vi "Adjust Font Size to Rectangle.vi"(7 "String Control Reference":refnum<vi>, 8 "Message":string, 9 "Bold?":bool, 10 "Maximum Size (45)":i16=45, 11 "Minimum Size (15)":i16=15) -> (3 "Font Size":u32)   [LabVIEW 2015, in "Test Class.lvclass"]
uses:
  Test Class.lvclass
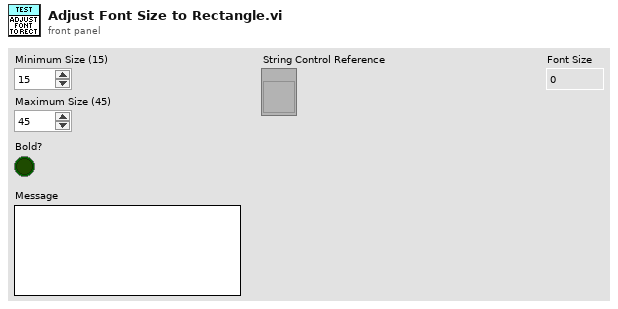
[diagram p1: front panel]
types:
  T1 = cluster{"Font Name:":string, "Size":i16, "Strikeout?":bool, "Italic?":bool, "Underline?":bool, "Outline?":bool, "Shadow?":bool, "Bold?":bool}
  T2 = enum16{"User-specified Font", "Application Font", "System Font", "Dialog Font"}
  T3 = cluster{"left":i16, "top":i16, "right":i16, "bottom":i16}
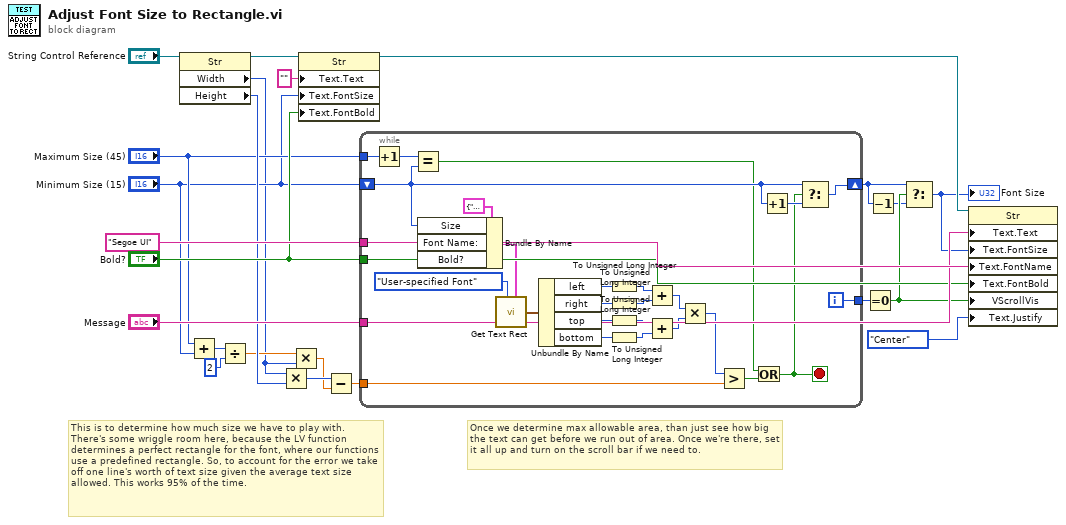
[diagram p0: block diagram]
diagram:
  w23 = "Segoe UI" ("Font Name:")
  # "Once we determine max allowable area, than just see how big the text can get before we run out of area. Once we're there, set it all up and turn on the scroll bar if we need to."
  # "This is to determine how much size we have to play with. There's some wriggle room here, because the LV function determines a perfect rectangle for the font, where our functions use a predefined rectangle. So, to account for the error we take off one line's worth of text size given the average text size allowed. This works 95% of the time."
  n1 = property on="Property Node" class="Str"(reference="String Control Reference") -> (reference out=w13:refnum<vi>, "Width"=w1:u32, "Height"=w11:u32)  [unwired: 1 in, 1 out]
  n2 = Add(x="Maximum Size (45)", y="Minimum Size (15)") -> (x+y=w6:i16)
  n3 = Divide(x=w6, y=i16 2) -> (x/y=w4:dbl)
  n4 = Multiply(x=w1, y=w11) -> (x*y=w18:u32)
  n5 = Multiply(x=w4, y=w1) -> (x*y=w17:dbl)
  n6 = property on="Property Node" class="Str"(reference=w13, "Text.Text"="", "Text.FontSize"="Minimum Size (15)", "Text.FontBold"="Bold?") -> (reference out=w12:refnum<vi>)  [unwired: 1 in, 1 out]
  n7 = Subtract(x=w18, y=w17) -> (x-y=w16:dbl)
  n8 = while {
    tunnel: "Message" -> [w50]
    tunnel: w23 -> [w48]
    tunnel: "Bold?" -> [w47]
    shift-right: [w30] -> w7
    shift-left: "Minimum Size (15)" -> [w28]
    tunnel: w16 -> [w41]
    tunnel: [w39] -> w22
    tunnel: "Maximum Size (45)" -> [w29]
    i -> [w39]
    stop <- w25 stop-if-true
    n9 = Increment(x=w29) -> (x+1=w24:i16)
    n10 = Equal?(x=w24, y=w28) -> (x = y?=w26:bool)
    n11 = Bundle By Name(cluster=T1 {"Font Name:"="Segoe UI", "Size"=0, "Strikeout?"=FALSE, "Italic?"=FALSE, "Underline?"=FALSE, "Outline?"=FALSE, "Shadow?"=FALSE, "Bold?"=FALSE} ("[user-specified font]"), "Size"=w28, "Font Name:"=w48, "Bold?"=w47) -> (w46:T1)
    n12 = call <vilib>:"Get Text Rect.vi"("desired font(Application)"=T2."User-specified Font", "text"=w50, "[user-specified font]"=w46) -> ("rect"=w45:T3)  [unwired: 6 in]
    n13 = Unbundle By Name(w45) -> ("left"=w44:i16, "right"=w38:i16, "top"=w37:i16, "bottom"=w36:i16)
    n14 = To Unsigned Long Integer(number=w44) -> (unsigned 32bit integer=w33:u32)
    n15 = To Unsigned Long Integer(number=w38) -> (unsigned 32bit integer=w32:u32)
    n16 = To Unsigned Long Integer(number=w37) -> (unsigned 32bit integer=w35:u32)
    n17 = To Unsigned Long Integer(number=w36) -> (unsigned 32bit integer=w34:u32)
    n18 = Add(x=w33, y=w32) -> (x+y=w42:u32)
    n19 = Add(x=w35, y=w34) -> (x+y=w43:u32)
    n20 = Multiply(x=w42, y=w43) -> (x*y=w40:u32)
    n21 = Greater?(x=w40, y=w41) -> (0:w27:bool)
    n22 = Or(x=w26, y=w27) -> (x .or. y?=w25:bool)
    n23 = Increment(x=w28) -> (x+1=w31:i16)
    n24 = Select(t=w28, s=w25, f=w31) -> (s? t:f=w30:i16)
  }
  n25 = Equal To 0?(x=w22) -> (x = 0?=w9:bool)
  n26 = Decrement(x=w7) -> (x-1=w8:i16)
  n27 = Select(t=w7, s=w9, f=w8) -> (s? t:f=w10:i16)
  "Font Size" <- w10
  n28 = property on="Property Node" class="Str"(reference=w12, "Text.Text"="Message", "Text.FontSize"=w10, "Text.FontName"=w23, "Text.FontBold"="Bold?", "VScrollVis"=w9, "Text.Justify"=enum16{"Left", "Center", "Right"}."Center" ("Text.Justification")) -> ()  [unwired: 1 in, 2 out]
